vi "InitializeItemContents.vi"(7 "separate test?":bool, 8 "error in (no error)":errorcluster, 10 "Root path":path, 11 "CLabVIEWItem in":refnum<class "CLabVIEWItem.lvclass">) -> (0 "error out":errorcluster, 3 "CLabVIEWItem out":refnum<class "CLabVIEWItem.lvclass">)   [LabVIEW 2020, in "LabVIEWItem.lvlib" / "CLabVIEWItem.lvclass"]
uses:
  CLabVIEWItem.lvclass
  CLabVIEWItem.lvclass/CLabVIEWItem.ctl
  <vilib>/regexp/Match Regular Expression.xnode
  CommonHelpers/CommonHelpers.lvlib
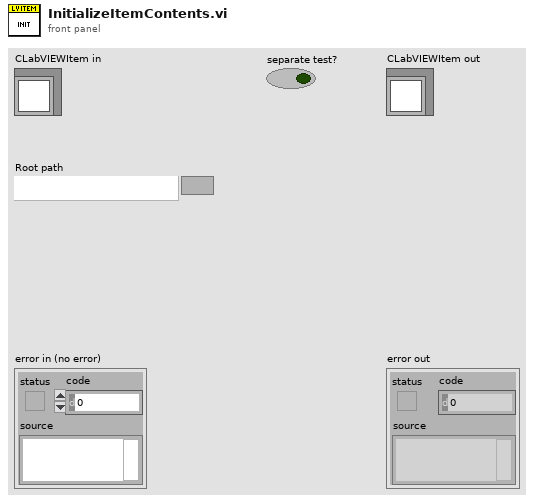
[diagram p1: front panel]
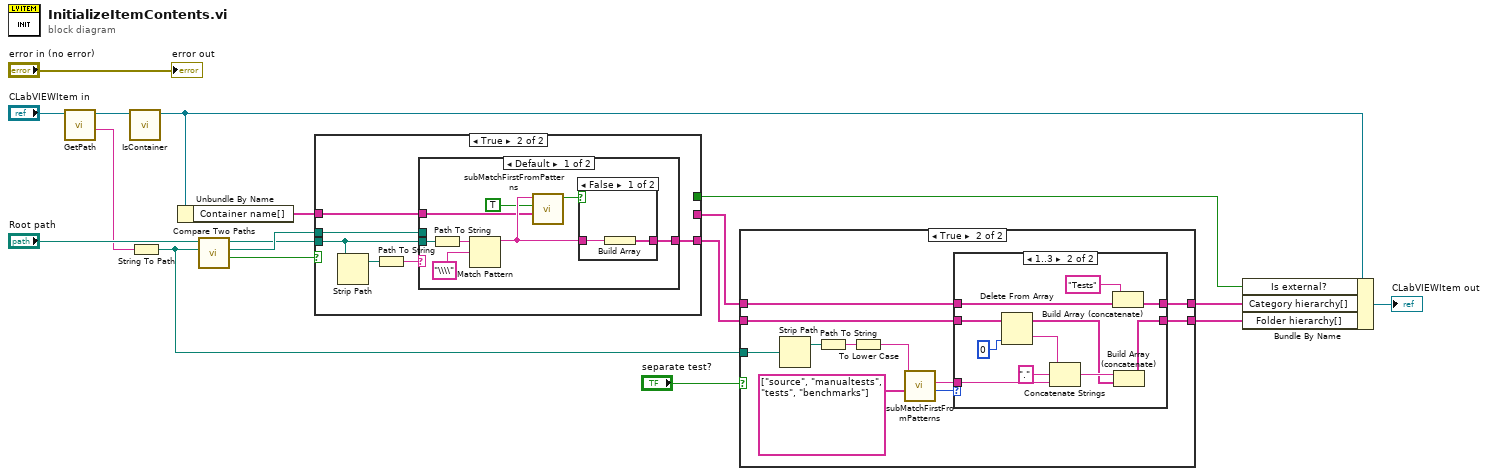
[diagram p0: block diagram]
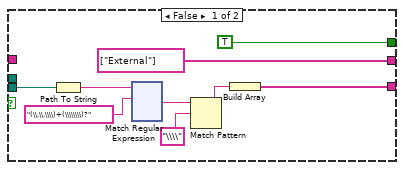
[diagram p2: hidden frame]
diagram:
  n1 = call-dynamic "GetPath.vi"("CLabVIEWItem in"="CLabVIEWItem in") -> ("Path"=w2:string, "CLabVIEWItem out"=w4:refnum<class "CLabVIEWItem.lvclass">)  [unwired: 8 in, 1 out]
  n2 = call-dynamic "IsContainer.vi"("CLabVIEWItem in"=w4) -> ("CLabVIEWItem out"=w3:refnum<class "CLabVIEWItem.lvclass">)  [unwired: 8 in, 2 out]
  n3 = String To Path(string=w2) -> (path=w1:path)
  n4 = Unbundle By Name(w3) -> ("Container name[]"=w5:string[])
  n5 = call <vilib>:"Compare Two Paths.vi"("Path 2"=w1, "Path 1"="Root path") -> ("Path 2 Relative to Path 1?"=w16:bool, "Common Path"=w18:path, "Relative Path from 1 to 2"=w17:path)  [unwired: 6 in, 1 out]
  n6 = case shown="True" w16 {
    tunnel: [w20 w143] -> w14
    tunnel: w17 -> [w27 w146]
    tunnel: w18 -> [_ w147]
    tunnel: [string[] ["External"] _] -> w15
    tunnel: [TRUE _] -> w7
    tunnel: w5 -> [_ w142]
    frame False {
      n7 = Path To String(path=w27) -> (string=w22:string)
      n8 = xnode "Match Regular Expression"("input string"=w22, "regular expression"="(\\.\\.\\\\)+(\\\\\\\\)?") -> ("after match"=w23:string)  [unwired: 4 in, 4 out]
      n9 = Match Pattern(string=w23, regular expression="\\\\") -> (before substring=w21:string)  [unwired: 1 in, 3 out]
      n10 = Build Array(w21) -> (w20:string[])
    }
    frame True {
      n11 = Strip Path(path=w146) -> (stripped path=w145:path)  [unwired: 1 out]
      n12 = Path To String(path=w145) -> (string=w144:string)
      n13 = case shown="Default" w144 {
        tunnel: w146 -> [w154 _]
        tunnel: [w152 _] -> w143
        tunnel: w147 -> [_ _]
        tunnel: w142 -> [w150 _]
        frame Default {
          n14 = Path To String(path=w154) -> (string=w153:string)
          n15 = Match Pattern(string=w153, regular expression="\\\\") -> (before substring=w151:string)  [unwired: 1 in, 3 out]
          n16 = call "subMatchFirstFromPatterns.vi"("patterns"=w150, "exact match?"=TRUE, "string in"=w151) -> ("found?"=w148:bool)  [unwired: 6 in, 2 out]
          n17 = case shown="False" w148 {
            tunnel: [w157 _] -> w152
            tunnel: w151 -> [w156 _]
            frame False {
              n18 = Build Array(w156) -> (w157:string[])
            }
            frame True {
            }
          }
        }
        frame "." {
        }
      }
    }
  }
  n19 = case shown="True" "separate test?" {
    tunnel: w1 -> [_ w170]
    tunnel: [w159 w164] -> w12
    tunnel: w15 -> [w158 w162]
    tunnel: w14 -> [w159 w161]
    tunnel: [w158 w160] -> w13
    frame False {
    }
    frame True {
      n20 = Strip Path(path=w170) -> (stripped path=w169:path)  [unwired: 1 out]
      n21 = Path To String(path=w169) -> (string=w168:string)
      n22 = To Lower Case(string=w168) -> (all lower case string=w167:string)
      n23 = call "subMatchFirstFromPatterns.vi"("patterns"=string[] ["source", "manualtests", "tests", "benchmarks"], "string in"=w167) -> ("index"=w166:i32, "matched string"=w165:string)  [unwired: 7 in, 1 out]
      n24 = case shown="1..3" w166 {
        tunnel: w161 -> [w172 w173]
        tunnel: [w172 w174] -> w164
        tunnel: w165 -> [_ w182]
        tunnel: w162 -> [w171 w180]
        tunnel: [w171 w179] -> w160
        frame 0, Default {
        }
        frame 1..3 {
          n25 = Delete From Array(array=w173, index=0) -> (deleted portion=w177:string, array with subset deleted=w175:string[])  [unwired: 1 in]
          n26 = Concatenate Strings(w177, "." ("string"), w182) -> (w176:string)
          n27 = Build Array (concatenate)("Tests" ("element"), w180) -> (w179:string[])
          n28 = Build Array (concatenate)(w176, w175) -> (w174:string[])
        }
      }
    }
  }
  n29 = Bundle By Name(cluster=w3, "Is external?"=w7, "Category hierarchy[]"=w13, "Folder hierarchy[]"=w12) -> (→"CLabVIEWItem out":refnum<class "CLabVIEWItem.lvclass">)
  "error out" <- "error in (no error)"
